vi "Configure Marker.vi"(5 "Marker Frequency (500 Hz)":dbl=500.0, 6 "Marker Cycle Number (2)":i32=2, 7 "Marker Pointer (10)":i32=10, 8 "error in (no error)":errorcluster, 9 "Marker Mode (0: Pointer)":i32(ring) items=["Pointer", "Frequency", "Cycle Number"], 10 "Source Channel (1: 1)":i32(ring)=1 items=["1"=1, "2"=2], 11 "VISA resource name":refnum<visa-resource-name>) -> (0 "error out":errorcluster, 3 "VISA resource name out":refnum<visa-resource-name>)   [LabVIEW 2026, in "Agilent 3352X Series.lvlib"]
doc: "Configures the point within an arbitrary waveform, sweep, or burst at which the front-panel Sync signal goes low."
uses:
  Agilent 3352X Series.lvlib
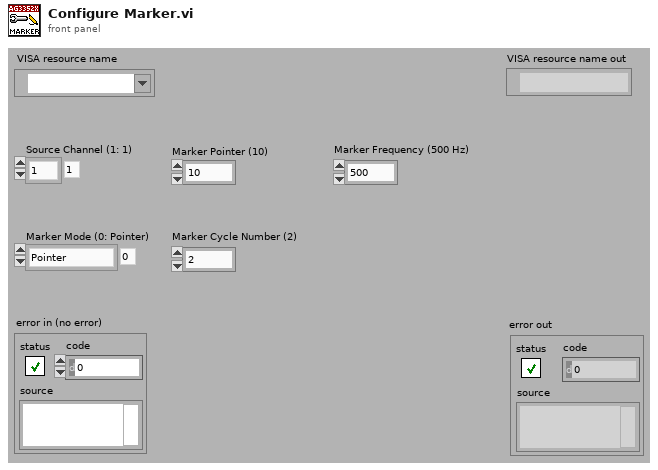
[diagram p1: front panel]
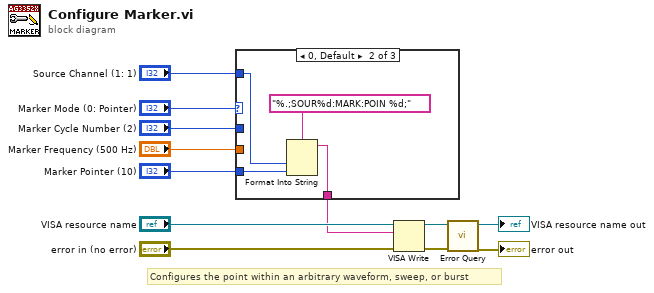
[diagram p0: block diagram]
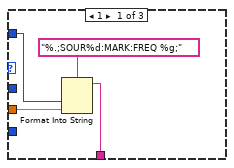
[diagram p2: hidden frame]
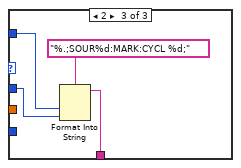
[diagram p3: hidden frame]
diagram:
  # "Configures the point within an arbitrary waveform, sweep, or burst"
  n1 = case shown="0, Default" "Marker Mode (0: Pointer)" {
    tunnel: [w16 w19 w23] -> w5
    tunnel: "Source Channel (1: 1)" -> [w14 w18 w22]
    tunnel: "Marker Frequency (500 Hz)" -> [w13 _ _]
    tunnel: "Marker Pointer (10)" -> [_ w17 _]
    tunnel: "Marker Cycle Number (2)" -> [_ _ w21]
    frame 1 {
      n2 = Format Into String(format string="%.;SOUR%d:MARK:FREQ %g;", w14, w13) -> (resulting string=w16:string)  [unwired: 2 in, 1 out]
    }
    frame 0, Default {
      n3 = Format Into String(format string="%.;SOUR%d:MARK:POIN %d;", w18, w17) -> (resulting string=w19:string)  [unwired: 2 in, 1 out]
    }
    frame 2 {
      n4 = Format Into String(format string="%.;SOUR%d:MARK:CYCL %d;", w22, w21) -> (resulting string=w23:string)  [unwired: 2 in, 1 out]
    }
  }
  n5 = VISA Write(VISA resource name="VISA resource name", write buffer=w5, error in (no error)="error in (no error)") -> (VISA resource name out=w10:refnum<visa-resource-name>, error out=w9:errorcluster)  [unwired: 1 out]
  n6 = call "Error Query.vi"("error in (no error)"=w9, "VISA resource name"=w10) -> ("error out"=→"error out":errorcluster, "VISA resource name out"=→"VISA resource name out":refnum<visa-resource-name>)  [unwired: 8 out]
